vi "Running Average.vi"(1 "New Value":dbl) -> (0 "Running Average":dbl)   [LabVIEW 2011]
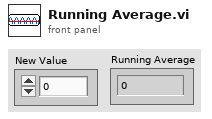
[diagram p1: front panel]
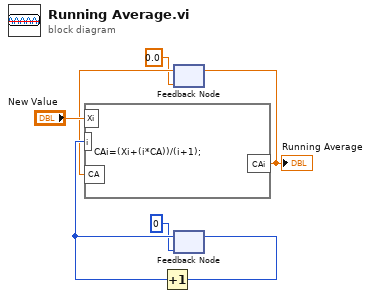
[diagram p0: block diagram]
diagram:
  n1 = feedback #1(0.0) -> (w3:dbl)
  n2 = feedback #2(u64 0) -> (w7:u64)
  n3 = formula code="CAi=(Xi+(i*CA))/(i+1);"("Xi"="New Value", "i"=w7, "CA"=w3) -> ("CAi"=w4:dbl)
  "Running Average" <- w4
  n4 = Increment(x=w7) -> (x+1=w6:u64)
  n5 = feedback-in #1(w4) -> ()
  n6 = feedback-in #2(w6) -> ()
